vi "rename_object.vi"(9 "label_visible":bool, 10 "new_label_name":string, 11 "id":string) -> (0 "error out":errorcluster)   [LabVIEW 2020]
doc: "Renames an objects label.text property, can be a control/indicator or a block diagram element like a constant."
uses:
  G-AI Core/G-AI Core.lvlib
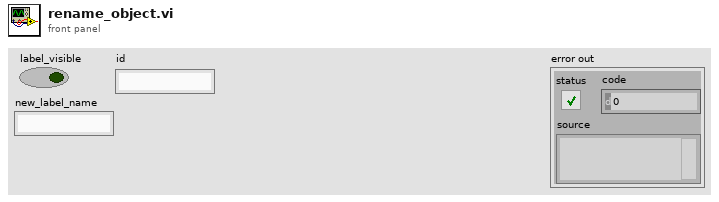
[diagram p1: front panel]
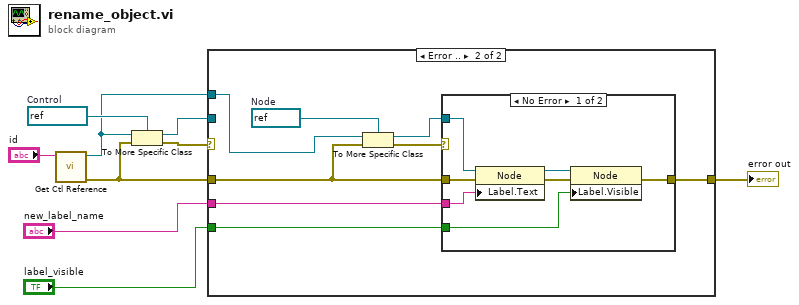
[diagram p0: block diagram]
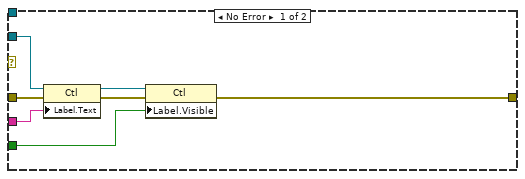
[diagram p2: hidden frame]
diagram:
  w8 = refnum<vi> refnum  # Control
  n1 = call "Get Ctl Reference.vi"("id"="id") -> ("error out"=w7:errorcluster, "ctl reference"=w6:refnum<vi>)  [unwired: 9 in]
  n2 = To More Specific Class(target class=w8, reference=w6, error in=w7) -> (specific class reference=w2:refnum<vi>, error out=w9:errorcluster)
  n3 = case shown="Error .." w9 {
    tunnel: w6 -> [_ w24]
    tunnel: "new_label_name" -> [w16 w18]
    tunnel: "label_visible" -> [w14 w19]
    tunnel: [w13 w22] -> w5
    tunnel: w7 -> [w11 w17]
    tunnel: w2 -> [w10 _]
    frame No Error {
      n4 = property class="Ctl"(reference=w10, error in=w11, "Label.Text"=w16) -> (reference out=w15:refnum<vi>, error out=w12:errorcluster)
      n5 = property class="Ctl"(reference=w15, error in=w12, "Label.Visible"=w14) -> (error out=w13:errorcluster)  [unwired: 1 out]
    }
    frame Error {
      w23 = refnum<vi> refnum  # Node
      n6 = To More Specific Class(target class=w23, reference=w24, error in=w17) -> (specific class reference=w20:refnum<vi>, error out=w21:errorcluster)
      n7 = case shown="No Error" w21 {
        tunnel: [w29 w32] -> w22
        tunnel: w20 -> [w30 _]
        tunnel: w19 -> [w27 _]
        tunnel: w18 -> [w26 _]
        tunnel: w17 -> [w25 w32]
        frame No Error {
          n8 = property class="Node"(reference=w30, error in=w25, "Label.Text"=w26) -> (reference out=w28:refnum<vi>, error out=w31:errorcluster)
          n9 = property class="Node"(reference=w28, error in=w31, "Label.Visible"=w27) -> (error out=w29:errorcluster)  [unwired: 1 out]
        }
        frame Error {
        }
      }
    }
  }
  "error out" <- w5
